vi "Unicode Input Example.vi"() -> ()   [LabVIEW 2020]
doc: "This example demonstrates unicode input with a string control."
uses:
  Types/Encoded UTF-8 String.ctl
  Unicode/Controls/String Encoding.ctl
  Types/UTF-8 String/UTF-8 String.lvclass/UTF-8 String.ctl
  Dialog & User Interface/Polymorphic VIs/Write Control Text/Write String Value (UTF-8 String).vi
  Dialog & User Interface/Polymorphic VIs/Read Control Text/Read String Value (UTF-8 String).vi
  Unicode/Encode String.vi
  Dialog & User Interface/Polymorphic VIs/Write Control Text/Write String Value (UTF-8 String).vi/5206cb6b-04fb-41f5-a37e-29c14f142303.vi
  Dialog & User Interface/Polymorphic VIs/Read Control Text/Read String Value (UTF-8 String).vi/bfba3187-b22e-4285-8cc2-1816a803f974.vi
  Private/Conversion/Text to UTF-8.vi
  Private/Conversion/Polymorphic VIs/Text to UTF-8 (LabVIEW String).vi
  Private/Conversion/Encoded UTF-8 String to Encoded UTF-16LE String.vi
  Private/Conversion/UTF-8 to Text.vi
  Private/Conversion/Polymorphic VIs/UTF-8 to Text (LabVIEW String).vi
  Private/Conversion/Encoded UTF-16LE String to Encoded UTF-8 String.vi
  Unicode/Prepend BOM.vi
  Private/Conversion/Text as Encoded String.vi
  Private/Conversion/Polymorphic VIs/Text as Encoded String (UTF-8 String).vi
  Unicode/SubVIs/Byte Order Marks.vi
  Unicode/Detect BOM.vi
  Types/UTF-8 String/Read Encoded UTF-8 String.vi
  Unicode/Detect String Encoding.vi
  Private/User Interface/Write String.vi
  Private/User Interface/Read String.vi
  Types/UTF-8 String/UTF-8 String.lvclass
  G-Unicode.lvlib
panel:
  out "Unicode Text":string
  in  "Unicode Input":string
  out "Value Change":string
  # "Instructions:\n1. Run the VI.\n2. Copy and paste some unicode text from Unicode Text into Unicode Input.\n3. Type some text into the Unicode Input control.\n4. Check the Value Change indicator matches the value in Unicode Input."
  # "Please note:\nWhile unicode input does work, LabVIEW's unicode input handling is experimental. You may observe text disappear from Unicode Input while typing, or the cursor doesn't match where text is being displayed as it is typed. This same behavior is present in NI's Unicode Toolkit in the Read Unicode from String Control.vi example."
  # "This example demonstrates unicode input handling.\n\nUnicode input to a string control requires the Force Unicode Text property to be enabled. Text typed into a string control which has this property enabled results in double-spaced characters (e.g. \"A B C \"). This occurs because the keyboard input is being processed as UTF-16LE unicode (2 bytes per char), but the text display assumes 1 byte per char.\n\nTo handle displaying typed unicode inputs, the string control must set the Interpret As Unicode property after every keystroke.\n\nTo manage these requirements, G-Unicode includes Update Unicode Controls.vi. This launches an asynchronous subVI which handles setting the appropriate unicode control properties, processing the keyboard inputs, and manages unicode display for the given string control references. It also provides a value change user event which can be registered, and is generated after the unicode updates are complete.\n\nNote that the asynchronous subVI must be terminated by generating an event on the Stop Event user event."
  # "G"
  # "-Unicode"
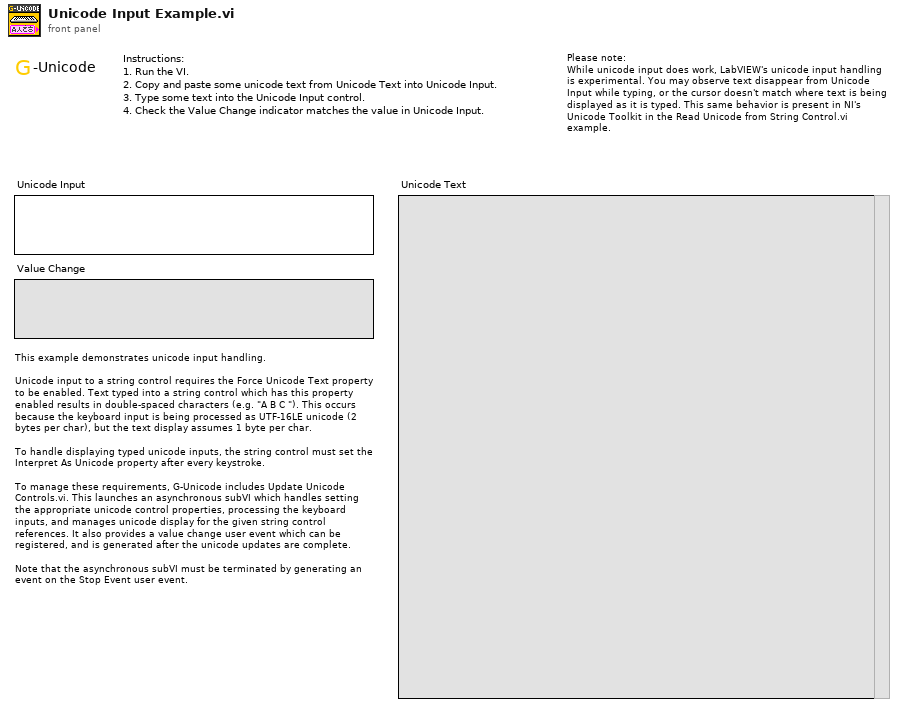
[diagram p1: front panel]
types:
  T1 = typedef "G-Unicode.lvlib/String Encoding.ctl" = enum16{"ANSI", "UTF-8", "UTF-16LE", "UTF-16BE", "Unknown"}
  T2 = typedef "G-Unicode.lvlib/Encoded UTF-8 String.ctl" = string
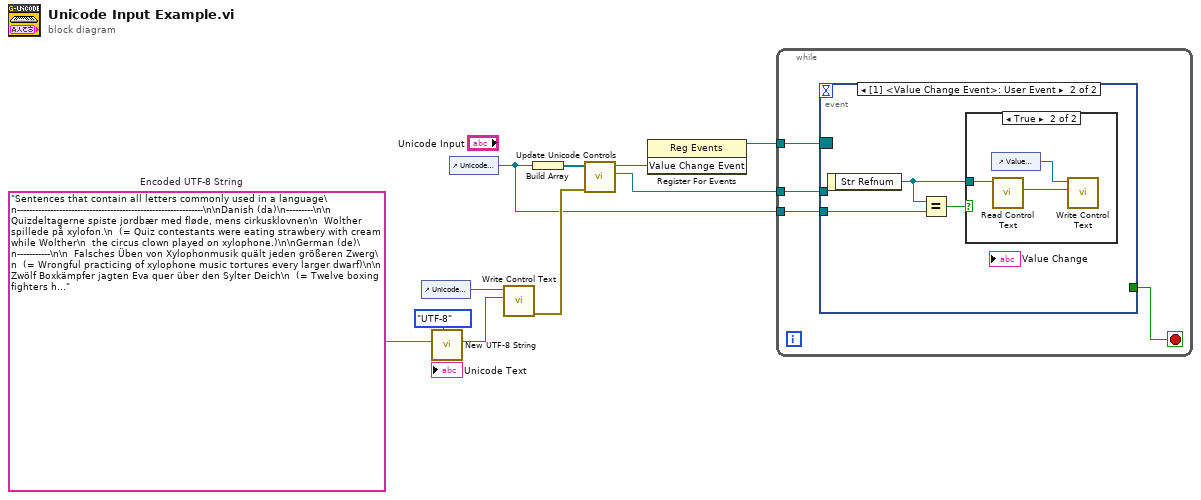
[diagram p0: block diagram]
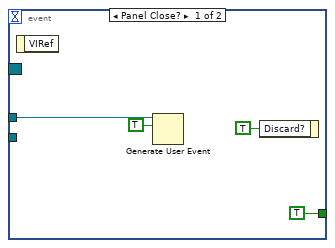
[diagram p2: hidden frame]
diagram:
  w3 = T2 "Sentences that contain all letters commonly used in a language\n--------------------------------------------------------------\n\nDanish (da)\n---------\n\n  Quizdeltagerne spiste jordbær med fløde, mens cirkusklovnen\n  Wolther spillede på xylofon.\n  (= Quiz contestants were eating strawbery with cream while Wolther\n  the circus clown played on xylophone.)\n\nGerman (de)\n-----------\n\n  Falsches Üben von Xylophonmusik quält jeden größeren Zwerg\n  (= Wrongful practicing of xylophone music tortures every larger dwarf)\n\n  Zwölf Boxkämpfer jagten Eva quer über den Sylter Deich\n  (= Twelve boxing fighters hunted Eva across the dike of Sylt)\n\n  Heizölrückstoßabdämpfung\n  (= fuel oil recoil absorber)\n  (jqvwxy missing, but all non-ASCII letters in one word)\n\nEnglish (en)\n------------\n\n  The quick brown fox jumps over the lazy dog\n\nSpanish (es)\n------------\n\n  El pingüino Wenceslao hizo kilómetros bajo exhaustiva lluvia y \n  frío, añoraba a su querido cachorro.\n  (Contains every letter and every accent, but not every combination\n  of vowel + acute.)\n\nFrench (fr)\n-----------\n\n  Portez ce vieux whisky au juge blond qui fume sur son île intérieure, à\n  côté de l'alcôve ovoïde, où les bûches se consument dans l'âtre, ce\n  qui lui permet de penser à la cænogenèse de l'être dont il est question\n  dans la cause ambiguë entendue à Moÿ, dans un capharnaüm qui,\n  pense-t-il, diminue çà et là la qualité de son œuvre. \n\n  l'île exiguë\n  Où l'obèse jury mûr\n  Fête l'haï volapük,\n  Âne ex aéquo au whist,\n  Ôtez ce vœu déçu.\n\n  Le cœur déçu mais l'âme plutôt naïve, Louÿs rêva de crapaüter en\n  canoë au delà des îles, près du mälström où brûlent les novæ.\n\nIrish Gaelic (ga)\n-----------------\n\n  D'fhuascail Íosa, Úrmhac na hÓighe Beannaithe, pór Éava agus Ádhaimh\n\nHungarian (hu)\n--------------\n\n  Árvíztűrő tükörfúrógép\n  (= flood-proof mirror-drilling machine, only all non-ASCII letters)\n\nIcelandic (is)\n--------------\n\n  Kæmi ný öxi hér ykist þjófum nú bæði víl og ádrepa\n\n  Sævör grét áðan því úlpan var ónýt\n  (some ASCII letters missing)\n\nJapanese (jp)\n-------------\n\n  Hiragana: (Iroha)\n\n  いろはにほへとちりぬるを\n  わかよたれそつねならむ\n  うゐのおくやまけふこえて\n  あさきゆめみしゑひもせす\n\n  Katakana:\n\n  イロハニホヘト チリヌルヲ ワカヨタレソ ツネナラム\n  ウヰノオクヤマ ケフコエテ アサキユメミシ ヱヒモセスン\n\nHebrew (iw)\n-----------\n\n  ? דג סקרן שט בים מאוכזב ולפתע מצא לו חברה איך הקליטה\n\nPolish (pl)\n-----------\n\n  Pchnąć w tę łódź jeża lub ośm skrzyń fig\n  (= To push a hedgehog or eight bins of figs in this boat)\n\nRussian (ru)\n------------\n\n  В чащах юга жил бы цитрус? Да, но фальшивый экземпляр!\n  (= Would a citrus live in the bushes of south? Yes, but only a fake one!)\n\nThai (th)\n---------\n\n  [--------------------------|------------------------]\n  ๏ เป็นมนุษย์สุดประเสริฐเลิศคุณค่า  กว่าบรรดาฝูงสัตว์เดรัจฉาน\n  จงฝ่าฟันพัฒนาวิชาการ           อย่าล้างผลาญฤๅเข่นฆ่าบีฑาใคร\n  ไม่ถือโทษโกรธแช่งซัดฮึดฮัดด่า     หัดอภัยเหมือนกีฬาอัชฌาสัย\n  ปฏิบัติประพฤติกฎกำหนดใจ        พูดจาให้จ๊ะๆ จ๋าๆ น่าฟังเอย ฯ\n\n  [The copyright for the Thai example is owned by The Computer\n  Association of Thailand under the Royal Patronage of His Majesty the\n  King.]\n"  # Encoded UTF-8 String
  n1 = control-ref of="Unicode Text"() -> (w7:refnum<vi>)
  n2 = call "New UTF-8 String.vi"("Input Encoding (ANSI)"=String_Encoding."UTF-8", "String"=w3) -> ("UTF-8 String"=w4:refnum<class "UTF-8 String.lvclass">)  [unwired: 8 in, 1 out]
  n3 = control-ref of="Unicode Input"() -> (w1:refnum<vi>)
  n4 = call-poly "Write Control Text.vi"("Value"=w4, "Control Ref"=w7) -> ("error out"=w6:errorcluster)  [unwired: 9 in]
  n5 = Build Array(w1) -> (w10:refnum<vi>[])
  n6 = call "Update Unicode Controls.vi"("error in"=w6, "String Refs"=w10) -> ("Stop Event"=w8:refnum<user-event>, "Value Change Event"=w2:refnum<user-event>)  [unwired: 7 in, 1 out]
  n7 = register-events(w2) -> (reference out=w9:refnum<event-registration>)  [unwired: 2 in, 1 out]
  n8 = while {
    tunnel: w9 -> [w14]
    tunnel: w1 -> [w13]
    tunnel: w8 -> [w12]
    stop <- w11 stop-if-true
    n9 = event shown="[1] <Value Change Event>: User Event" {
      selector: w14 -> [_ _]
      dyn-events: _ -> [_ _]
      timeout: _ -> [_ _]
      tunnel: w13 -> [_ w21]
      tunnel: w12 -> [w17 _]
      tunnel: [TRUE _] -> w11
      event Panel Close? {
        n10 = event-data() -> ()  [unwired: 1 in, 1 out]
        n11 = Generate User Event(user event=w17, event data cluster=TRUE ("event data")) -> ()  [unwired: 2 in, 2 out]
        n12 = event-data("Discard?"=TRUE) -> ()  [unwired: 1 in, 1 out]
      }
      event User Event {
        n13 = event-data() -> ("Str Refnum"=w19:refnum<vi>)  [unwired: 1 in]
        n14 = Equal?(x=w19, y=w21) -> (x = y?=w20:bool)
        n15 = case shown="True" w20 {
          tunnel: w19 -> [_ w24]
          frame False {
          }
          frame True {
            n16 = control-ref of="Value Change"() -> (w22:refnum<vi>)
            n17 = call-poly "Read Control Text.vi"("Control Ref"=w24) -> ("UTF-8 String"=w23:refnum<class "UTF-8 String.lvclass">)  [unwired: 9 in, 1 out]
            n18 = call-poly "Write Control Text.vi"("Value"=w23, "Control Ref"=w22) -> ()  [unwired: 9 in, 1 out]
          }
        }
      }
    }
  }
